vi "Test pulse integration in file.vi"(8 "Error In":errorcluster, 10 "group name in":string="Untitled", 11 "File Path Control":path=path "\\\\eden\\NHMFLDATA/Data/Generator/January_2016/012516/rp164348_012516.tdms") -> (0 "Error Out":errorcluster)   [LabVIEW 2015]
uses:
  Utilities/Controls/Integrate channel.ctl
panel:
  out "Integrated Waveform":waveform(dbl)
  out "Waveform Graph 2":waveform(dbl)(graph)
  in  "Save data":bool
  in  "Offset duration":dbl=0.1 format="%#_6p"
  in  "Integration settings":T1={"Channel"="CH0", "Output name"="Current", "Factor"=1.0, "Start time"=0.0, "Duration"=0.0} {"Duration" format="%#_6p"; "Start time" format="%#_6p"}
  out "Waveform Graph":waveform(dbl)(graph)
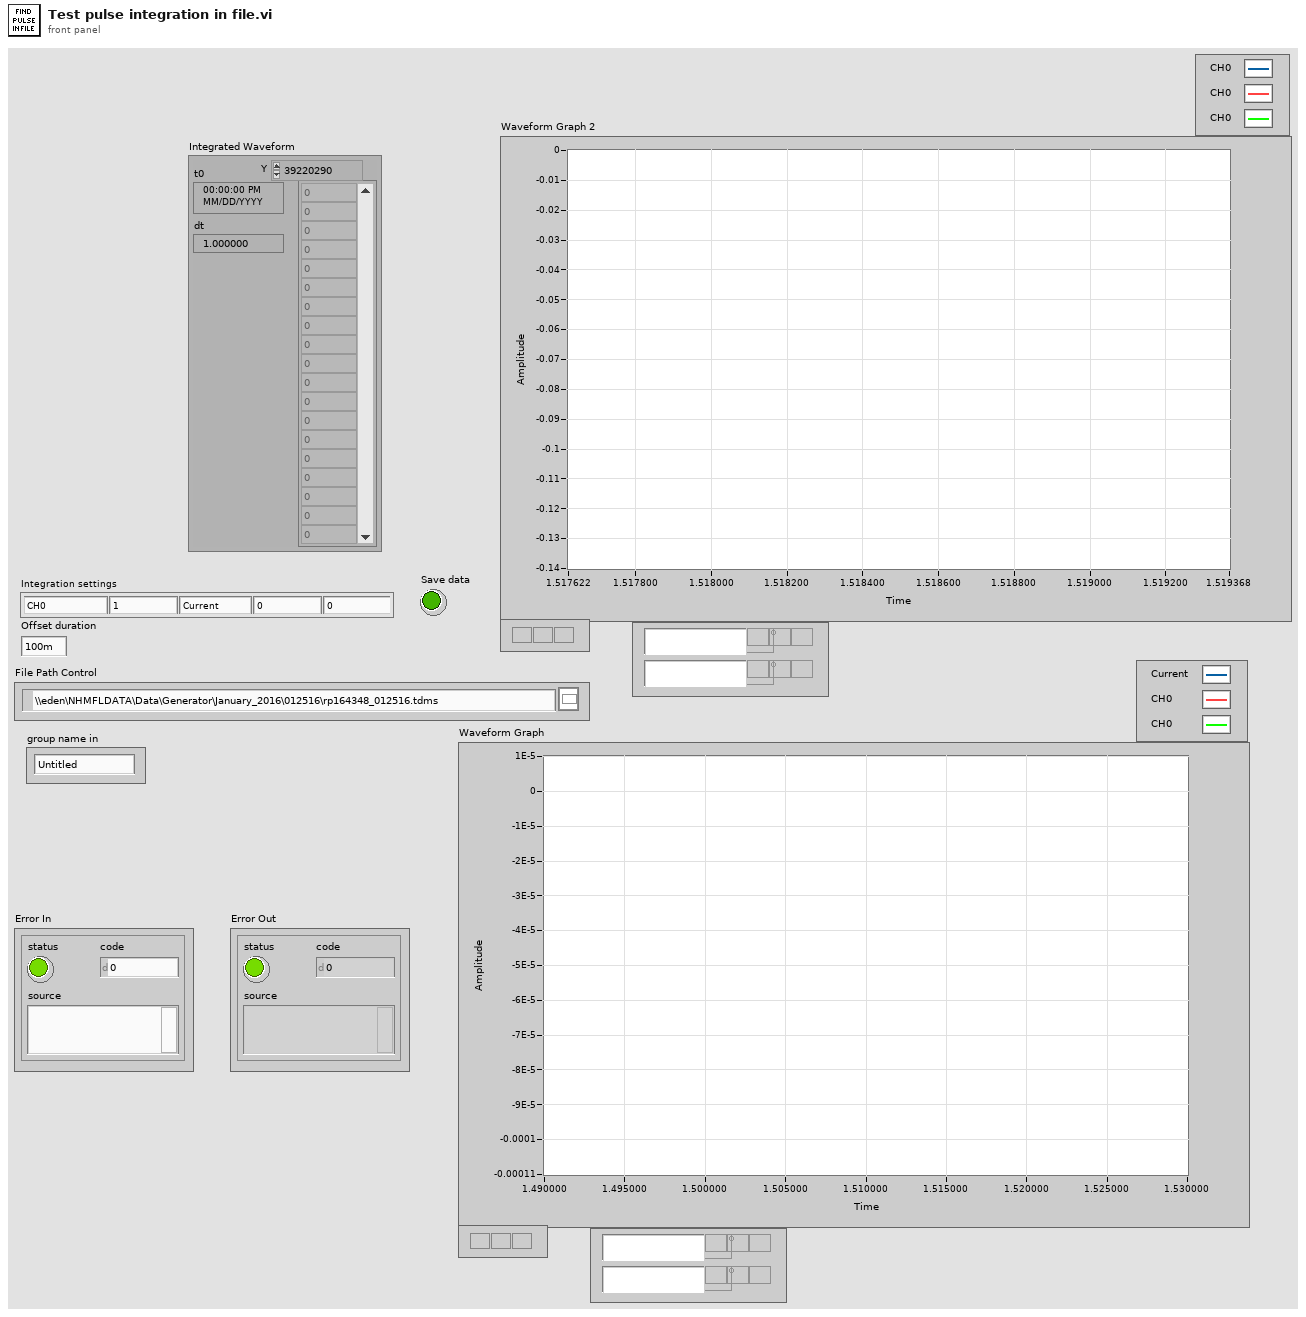
[diagram p1: front panel]
types:
  T1 = typedef "Integrate channel.ctl" = cluster{"Channel":string, "Output name":string, "Factor":dbl, "Start time":dbl, "Duration":dbl}
  T2 = enum16{"open", "open or create", "create or replace", "create", "open (read-only)"}
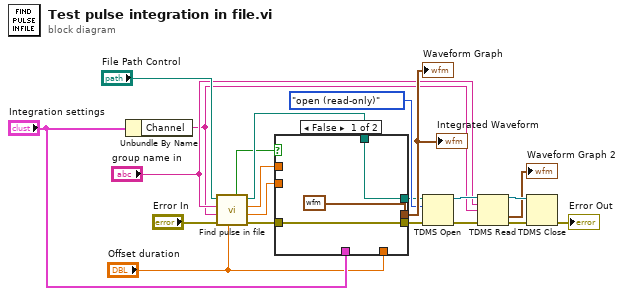
[diagram p0: block diagram]
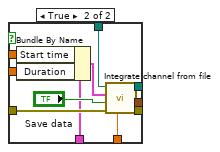
[diagram p2: hidden frame]
diagram:
  n1 = Unbundle By Name("Integration settings") -> ("Channel"=w5:string)
  n2 = call "Find pulse in file.vi"("Offset duration"="Offset duration", "Error In"="Error In", "Channel"=w5, "group name in"="group name in", "File Path Control"="File Path Control") -> ("Error Out"=w19:errorcluster, "duration"=w16:dbl, "Start time"=w17:dbl, "File Path out"=w18:path, "Found"=w1:bool)  [unwired: 2 in]
  n3 = case shown="False" w1 {
    tunnel: w19 -> [w24 w35]
    tunnel: w18 -> [w22 w34]
    tunnel: w17 -> [_ w32]
    tunnel: w16 -> [_ w31]
    tunnel: [waveform(dbl) {"t0"=timestamp(0 s since 1904-01-01), "dt"=1.0, "Y"=[]} ("Integrated Waveform") w30] -> w15
    tunnel: "Integration settings" -> [_ w28]
    tunnel: "Offset duration" -> [_ w27]
    tunnel: [w22 w26] -> w7
    tunnel: [w24 w25] -> w4
    frame False {
    }
    frame True {
      n4 = Bundle By Name(cluster=w28, "Start time"=w32, "Duration"=w31) -> (w33:T1)
      n5 = call "Integrate channel from file.vi"("Offset duration"=w27, "Error In"=w35, "Save data"="Save data", "Integration settings"=w33, "File Path Control"=w34) -> ("Error Out"=w25:errorcluster, "Integrated Waveform"=w30:waveform(dbl), "File Path out"=w26:path)  [unwired: 3 in, 1 out]
    }
  }
  "Waveform Graph" <- w15
  "Integrated Waveform" <- w15
  n6 = TDMS Open(8:w4, 10:T2."open (read-only)" ("operation (0:open)"), 11:w7) -> (0:w10:errorcluster, 3:w11:refnum<k34>)  [unwired: 4 in]
  n7 = TDMS Read(0:w11, 5:"group name in", 7:w5, 11:w10) -> (4:w9:refnum<k34>, 10:→"Waveform Graph 2":waveform(dbl), 15:w8:errorcluster)  [unwired: 4 in, 3 out]
  n8 = TDMS Close(8:w8, 11:w9) -> (0:→"Error Out":errorcluster)  [unwired: 1 out]
